vi "Example-Target.vi"   [LabVIEW 2018]
types:
  T1 = cluster{"API":cluster{"R&R Enqueuer":refnum<user-event>}, "Something Else":string}
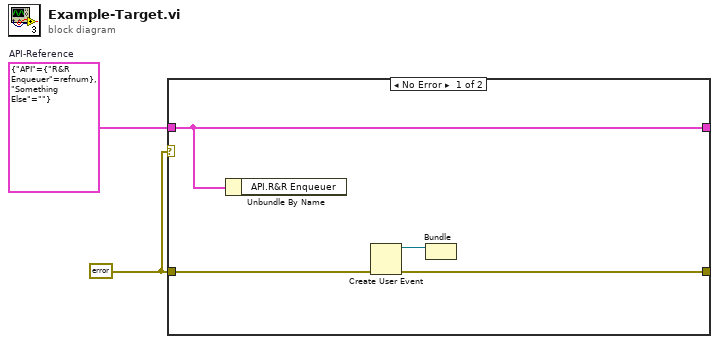
[diagram p0: block diagram]
diagram:
  w1 = errorcluster {"status"=FALSE, "code"=0, "source"=""} ("error IO")
  w2 = T1 {"API"={"R&R Enqueuer"=refnum}, "Something Else"=""}  # API-Reference
  n1 = case shown="No Error" w1 {
    selector: w1 -> [_ w8]
    tunnel: w2 -> [w6 w7]
    tunnel: [w6 w7] -> _
    tunnel: w1 -> [w5 _]
    tunnel: [w3 w8] -> _
    frame No Error {
      n2 = Unbundle By Name(w6) -> ()  [unwired: 1 out]
      n3 = Create User Event(error in=w5) -> (user event=w4:refnum<user-event>, error out=w3:errorcluster)  [unwired: 1 in]
      n4 = Bundle("Stopped"=w4) -> ()  [unwired: 2 in, 1 out]
    }
    frame Error {
    }
  }
